vi "sub_MFSKMod.vi"(6 "filter parameters":T2={"Alpha"=0.5, "Filter Length"=6, "TX Filter"=enum."Root Raised Cos"} {"Alpha" format="%.2f"}, 8 "Symbol Rate, Hz":dbl=1.0 format="%.2f", 9 "Packet to Transmit":i8[](array[numeric]), 10 "FSK system parameters":T1 {"symbol map" format="%.2f"}) -> (2 "output complex waveform":cluster{"t0":dbl, "dt":dbl, "Y":cdb[]} {"Y" format="%.3f"; "dt" format="%^.2e"; "t0" format="%.4f"})   [LabVIEW 2015]
uses:
  <vilib>/addons/Modulation/Digital/Support/Controls/FSK System Parameters.ctl
  <vilib>/addons/Modulation/Analog/support/mod_Set Error Source.vi
  <vilib>/addons/Modulation/Digital/Support/Common/Validators/mod_Generate Filter Coefficients Validate.vi
  <vilib>/addons/Modulation/Digital/General/subVIs/mod_Generate Filter Coefficients.vi
  <vilib>/addons/Modulation/niDMT.lvlib
panel:
  out "error out":errorcluster
  in  "error in (no error)":errorcluster
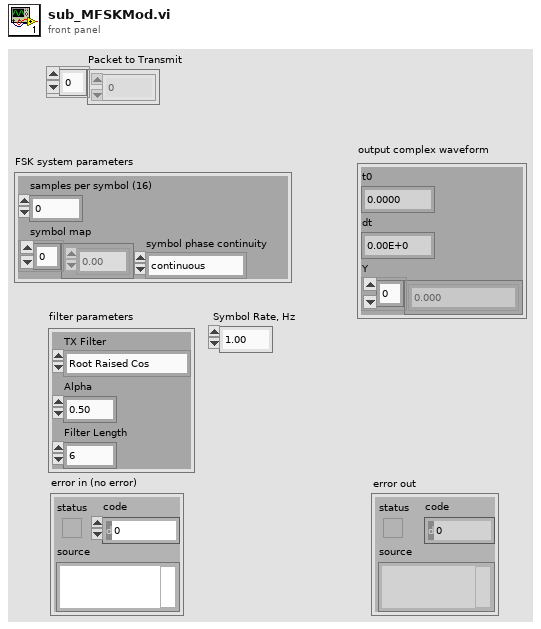
[diagram p1: front panel]
types:
  T1 = typedef "niDMT.lvlib/FSK System Parameters.ctl" = cluster{"samples per symbol (16)":i32, "symbol map":dbl[], "symbol phase continuity":enum16{"continuous", "discontinuous"}}
  T2 = cluster{"Alpha":dbl, "Filter Length":i32, "TX Filter":enum16{"none", "Raised Cosine", "Root Raised Cos", "Gaussian"}}
  T3 = enum16{"FSK", "PSK", "QAM", "MSK", "PAM", "ASK", "CPM"}
  T4 = enum16{"none", "Raised Cosine", "Root Raised Cos", "Gaussian"}
  T5 = typedef "niAMT.lvlib/Complex Data Waveform.ctl" = cluster{"t0":dbl, "dt":dbl, "Y":cdb[]}
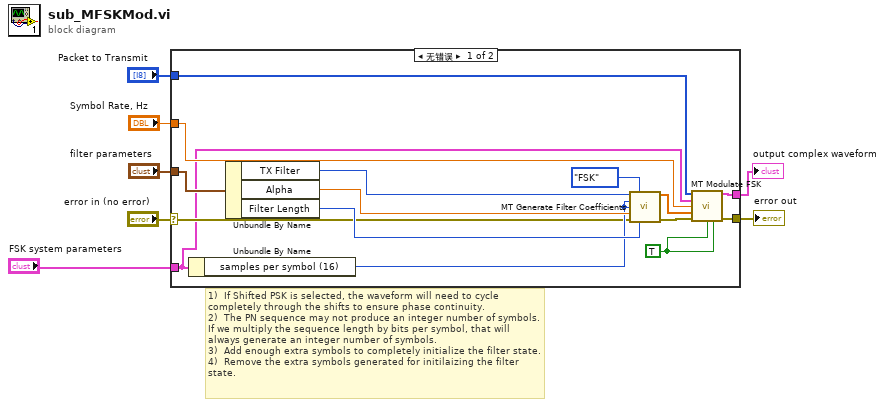
[diagram p0: block diagram]
diagram:
  # "1)  If Shifted PSK is selected, the waveform will need to cycle completely through the shifts to ensure phase continuity. \n2)  The PN sequence may not produce an integer number of symbols.  If we multiply the sequence length by bits per symbol, that will always generate an integer number of symbols. \n3)  Add enough extra symbols to completely initialize the filter state.\n4)  Remove the extra symbols generated for initilaizing the filter state."
  n1 = case shown="无错误" "error in (no error)" {
    selector: "error in (no error)" -> [w10 w23]
    tunnel: [w13 _] -> w7
    tunnel: [w22 w23] -> w6
    tunnel: "Symbol Rate, Hz" -> [w19 _]
    tunnel: "FSK system parameters" -> [w8 _]
    tunnel: "filter parameters" -> [w12 _]
    tunnel: "Packet to Transmit" -> [w14 _]
    frame No Error {
      w9 = TRUE ("Reset (T)")
      n2 = Unbundle By Name(w8) -> ("samples per symbol (16)"=w15:i32)
      n3 = Unbundle By Name(w12) -> ("TX Filter"=w20:T4, "Alpha"=w21:dbl, "Filter Length"=w17:i32)
      n4 = call <vilib>:"MT Generate Filter Coefficients.vi"("pulse shaping filter (none)"=w20, "modulation type"=T3."FSK", "pulse shaping samples per symbol (16)"=w15, "matched samples per symbol (16)"=w15, "filter parameter"=w21, "error in (no error)"=w10, "filter length (symbols)"=w17) -> ("pulse shaping filter coefficients"=w18:dbl[], "error out"=w16:errorcluster)  [unwired: 6 in, 1 out]
      n5 = call <vilib>:"MT Modulate FSK.vi"("input bit stream"=w14, "FSK system parameters"=w8, "symbol rate (Hz)"=w19, "pulse shaping filter coefficients"=w18, "error in (no error)"=w16, "reset? (T)"=w9, "flush buffers? (F)"=w9) -> ("output complex waveform"=w13:T5, "error out"=w22:errorcluster)  [unwired: 5 in, 2 out]
    }
    frame Error {
    }
  }
  "error out" <- w6
  "output complex waveform" <- w7
